vi "Steuerung kommunizieren.vi"(0 "Steuerung PNS Eingang":refnum<class "Steuerung PNS.lvclass">, 1 "Adressen":T1, 2 "Werte":T2, 3 "error in (no error)":errorcluster caption="Fehler (Eingang, kein Fehler)") -> (7 "Steuerung PNS Ausgang":refnum<class "Steuerung PNS.lvclass">, 8 "Istwerte":u16[](array[numeric]), 10 "error out":errorcluster caption="Fehler (Ausgang)")   [LabVIEW 2020, in "Steuerung PNS.lvclass"]
doc: "Low Level Kommunikation mit der Steuerung.\nLesen auf den Adressen vom Input und Schreiben der Werte vom Input.\nGibt die Istwerte als Output zurück (diese wurden im Lesen bereits im Objekt gesichert).\nRIW"
uses:
  Steuerung PNS.lvclass
  Werte.ctl
  Adresse.ctl
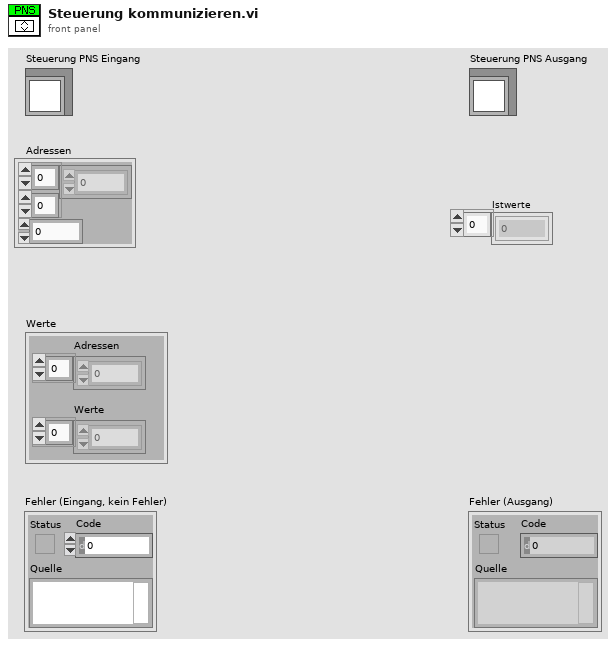
[diagram p1: front panel]
types:
  T1 = typedef "Steuerung PNS.lvclass/Adresse.ctl" = cluster{i32[][], i32}
  T2 = typedef "Steuerung PNS.lvclass/Werte.ctl" = cluster{"Adressen":u16[], "Werte":u16[]}
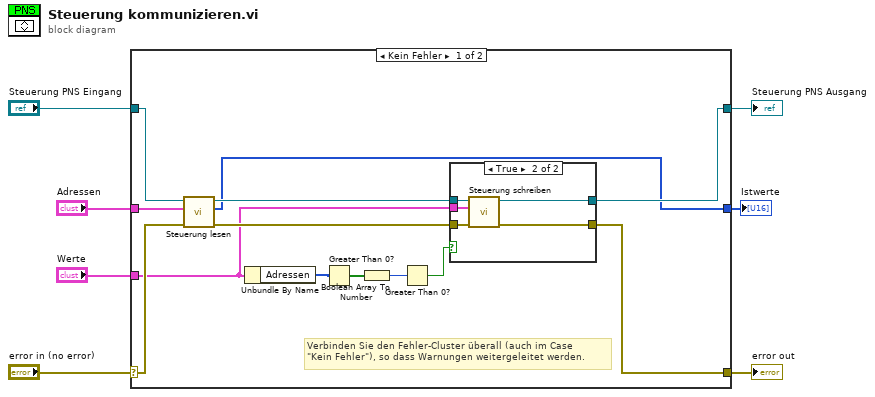
[diagram p0: block diagram]
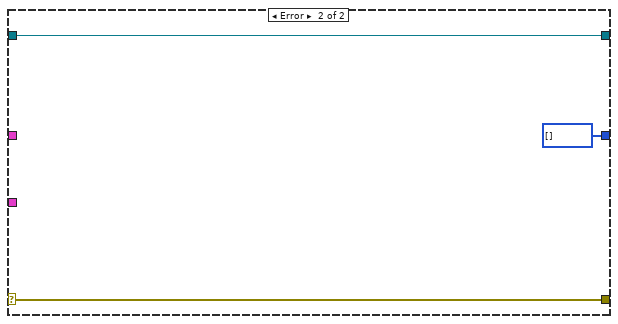
[diagram p3: hidden frame]
diagram:
  n1 = case shown="Kein Fehler" "error in (no error)" {
    selector: "error in (no error)" -> [w18 w30]
    tunnel: [w17 w30] -> w6
    tunnel: [w9 w29] -> w4
    tunnel: "Steuerung PNS Eingang" -> [w20 w29]
    tunnel: "Adressen" -> [w16 _]
    tunnel: "Werte" -> [w14 _]
    tunnel: [w8 u16[] [] ("Istwerte")] -> w1
    frame No Error {
      # "Verbinden Sie den Fehler-Cluster überall (auch im Case\n\"Kein Fehler\"), so dass Warnungen weitergeleitet werden."
      n2 = call "Steuerung lesen.vi"("Steuerung PNS Eingang"=w20, "Adressen"=w16, "error in (no error)"=w18) -> ("Steuerung PNS Ausgang"=w15:refnum<class "Steuerung PNS.lvclass">, "Istwerte"=w8:u16[], "error out"=w19:errorcluster)  [unwired: 5 in]
      n3 = Unbundle By Name(w14) -> ("Adressen"=w13:u16[])
      n4 = Greater Than 0?(x=w13) -> (x > 0?=w12:bool[])
      n5 = Boolean Array To Number(Boolean array=w12) -> (number=w11:u32)
      n6 = Greater Than 0?(x=w11) -> (x > 0?=w10:bool)
      n7 = case shown="True" w10 {
        tunnel: w19 -> [w22 w27]
        tunnel: [w22 w26] -> w17
        tunnel: w15 -> [w21 w25]
        tunnel: w14 -> [_ w24]
        tunnel: [w21 w23] -> w9
        frame False {
        }
        frame True {
          n8 = call "Steuerung schreiben.vi"("error in (no error)"=w27, "Werte"=w24, "Steuerung PNS Eingang"=w25) -> ("error out"=w26:errorcluster, "Steuerung PNS Ausgang"=w23:refnum<class "Steuerung PNS.lvclass">)  [unwired: 7 in]
        }
      }
    }
    frame Error {
    }
  }
  "error out" <- w6
  "Steuerung PNS Ausgang" <- w4
  "Istwerte" <- w1
